vi "Test Test Pass if Expected Error Throwm.vi"(8 "error in (no error)":errorcluster, 11 "Test Case In":refnum<class "Pure Mock One Expectation Test.lvclass">) -> (0 "error out":errorcluster, 3 "Test Case Out":refnum<class "Pure Mock One Expectation Test.lvclass">)   [LabVIEW 2020, in "Pure Mock One Expectation Test.lvclass"]
uses:
  Pure Mock One Expectation Test.lvclass
  C:/Program Files (x86)/National Instruments/LabVIEW 2020/vi.lib/Astemes/LUnit/Test Case.lvclass
  Test Doubles/Test Interface Pure Mock/Test Interface Pure Mock.lvclass
  C:/git/astemes-lmock/source/Core/Mock/Mock.lvclass
  source/Expectations/One/One.lvclass
  Expectation Test/Responsive Mock Expectation Test.lvclass
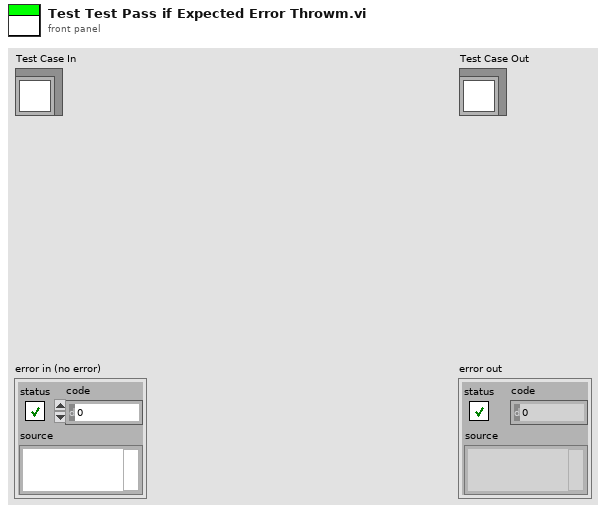
[diagram p1: front panel]
types:
  T1 = enum16{"", "Passed", "Failed", "Error", "Skipped", "Setup Error", "Broken", "Teardown Error"}
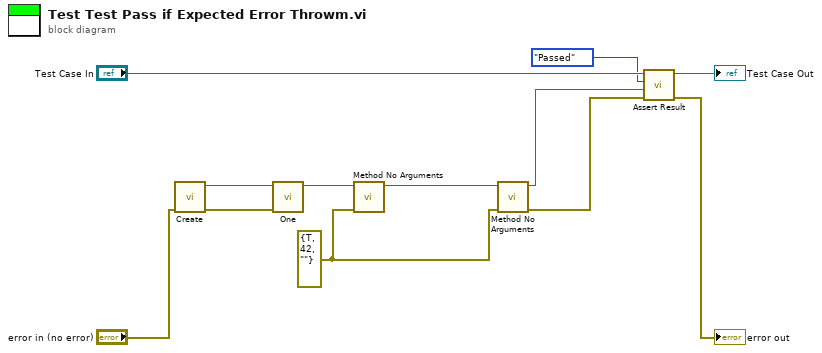
[diagram p0: block diagram]
diagram:
  w1 = errorcluster {"status"=TRUE, "code"=42, "source"=""} ("error in (no error)")
  n1 = call "Create.vi"("error in (no error)"="error in (no error)") -> ("error out"=w11:errorcluster, "Test Interface Mock Out"=w12:refnum<class "Test Interface Pure Mock.lvclass">)  [unwired: 9 in]
  n2 = call "One.vi"("error in (no error)"=w11, "Mock in"=w12) -> ("Mock out"=w10:refnum<class "Test Interface Pure Mock.lvclass">)  [unwired: 8 in, 1 out]
  n3 = call-dynamic "Method No Arguments.vi"("error in (no error)"=w1, "Mock In"=w10) -> ("Mock Out"=w3:refnum<class "Test Interface Pure Mock.lvclass">)  [unwired: 8 in, 1 out]
  n4 = call-dynamic "Method No Arguments.vi"("error in (no error)"=w1, "Mock In"=w3) -> ("error out"=w4:errorcluster, "Mock Out"=w2:refnum<class "Test Interface Pure Mock.lvclass">)  [unwired: 8 in]
  n5 = call "Assert Result.vi"("error in (no error)"=w4, "Mock"=w2, "Status"=T1."Passed", "LUnit Test Case In"="Test Case In") -> ("error out"=→"error out":errorcluster, "LUnit Test Case Out"=→"Test Case Out":refnum<class "Pure Mock One Expectation Test.lvclass">)  [unwired: 6 in]
